vi "INIgetSection.vi"(10 "SectionName":string, 11 "INIfilePath":path) -> (0 "Error Out":errorcluster, 1 "SectionValues":string[](array[string]), 2 "SectionKeys":string[](array[string]), 3 "key-ValArray":cluster{"key":string, "value":string}[](array[cluster]))   [LabVIEW 2021]
uses:
  <vilib>/Utility/config.llb/Read Key (String).vi
  <vilib>/Utility/config.llb/NI_LVConfig.lvlib
panel:
  in  "Error In":errorcluster
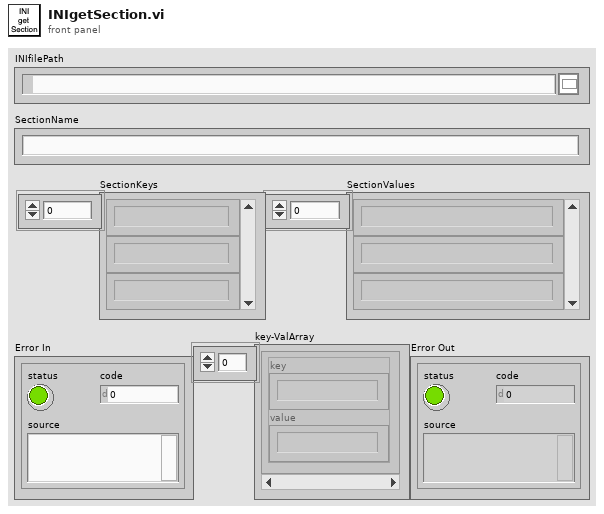
[diagram p1: front panel]
types:
  T1 = typedef "NI_LVConfig.lvlib/Config Data RefNum.ctl" = refnum<k1>
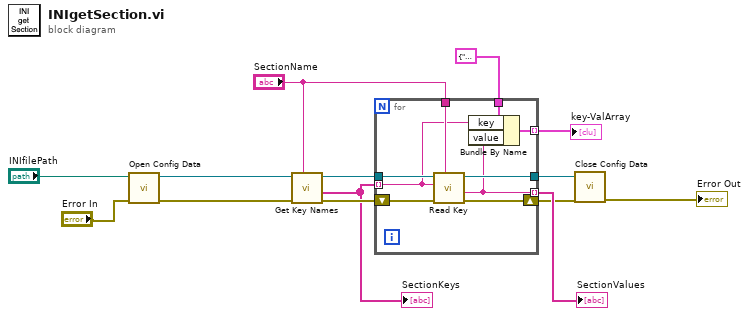
[diagram p0: block diagram]
diagram:
  n1 = call <vilib>:"Open Config Data.vi"("error in (no error)"="Error In", "configuration file path"="INIfilePath") -> ("error out"=w12:errorcluster, "refnum"=w14:T1)  [unwired: 7 in, 1 out]
  n2 = call <vilib>:"Get Key Names.vi"("section"="SectionName", "error in (no error)"=w12, "refnum"=w14) -> ("error out"=w6:errorcluster, "key names"=w3:string[], "refnum out"=w10:T1)  [unwired: 5 in, 1 out]
  "SectionKeys" <- w3
  n3 = for {
    tunnel: "SectionName" -> [w21]
    tunnel: w3 -> [w17] mode=indexing
    tunnel: w10 -> [w23]
    tunnel: [w22] -> w9
    tunnel: [w16] -> w7 mode=indexing
    shift-right: [w19] -> w5
    shift-left: w6 -> [w20]
    tunnel: cluster{"key":string, "value":string} {"key"="", "value"=""} -> [w18]
    tunnel: [w15] -> w1 mode=indexing
    n4 = call-poly <vilib>:"Read Key.vi"("section"=w21, "error in (no error)"=w20, "key"=w17, "refnum"=w23) -> ("error out"=w19:errorcluster, "value"=w16:string, "refnum out"=w22:T1)  [unwired: 4 in, 1 out]
    n5 = Bundle By Name(cluster=w18, "key"=w17, "value"=w16) -> (w15:cluster{"key":string, "value":string})
  }
  "SectionValues" <- w7
  "key-ValArray" <- w1
  n6 = call <vilib>:"Close Config Data.vi"("error in (no error)"=w5, "refnum"=w9) -> ("error out"=→"Error Out":errorcluster)  [unwired: 8 in, 1 out]
